vi "Generate Process.vi"(8 "error in (no error)":errorcluster, 9 "Directory":path, 10 "Name":string, 11 "Process Generator In":refnum<class "Process Generator.lvclass">) -> (0 "error out":errorcluster, 3 "Process Generator Out":refnum<class "Process Generator.lvclass">)   [LabVIEW 2020, in "Process Generator.lvclass"]
uses:
  Process Generator.lvclass
  Process Generator.lvclass/Process Generator.ctl
  Framework/Process/Process.lvclass
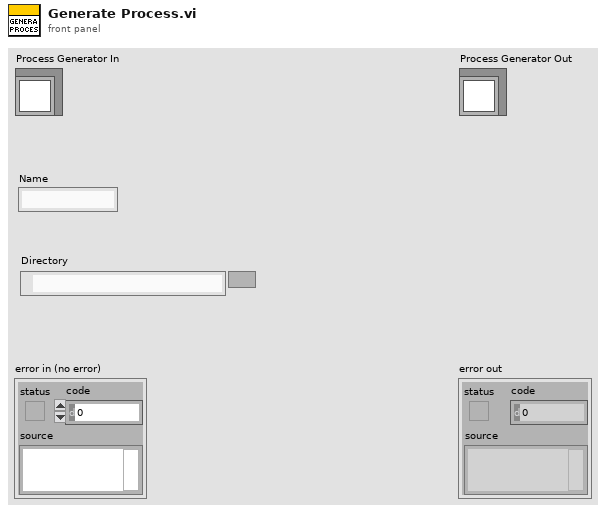
[diagram p1: front panel]
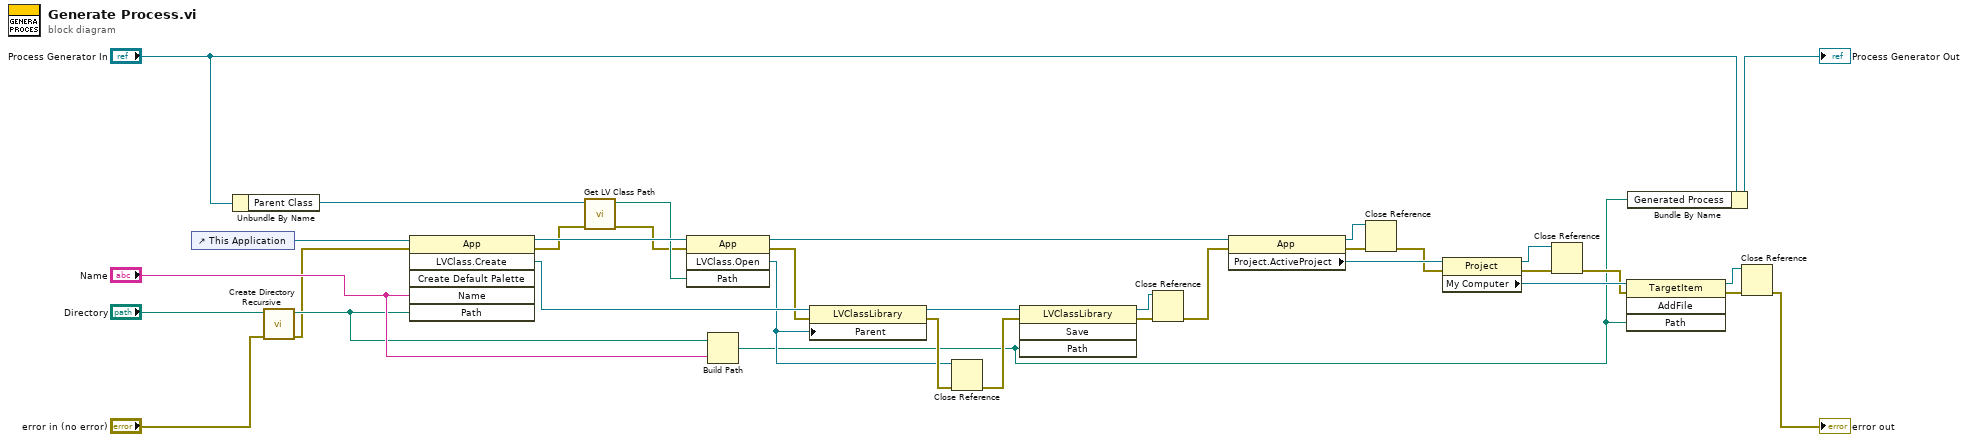
[diagram p0: block diagram]
diagram:
  n1 = control-ref of="This Application"() -> (w1:refnum<vi>)
  n2 = Unbundle By Name("Process Generator In") -> ("Parent Class"=w33:refnum<class "Process.lvclass">)
  n3 = call <vilib>:"Create Directory Recursive.vi"("error in (no error)"="error in (no error)", "directory"="Directory") -> ("error out"=w15:errorcluster, "directory copy"=w17:path)  [unwired: 3 in, 1 out]
  n4 = invoke class="App" method="LVClass.Create"(reference=w1, error in=w15, "Name"="Name", "Path"=w17) -> (reference out=w32:refnum<vi>, error out=w14:errorcluster, "LVClass.Create"=w35:refnum<vi>)  [unwired: 2 in, 3 out]
  n5 = call <vilib>:"Get LV Class Path.vi"("error in (no error)"=w14, "object"=w33) -> ("error out"=w13:errorcluster, "class path"=w31:path)  [unwired: 8 in]
  n6 = invoke class="App" method="LVClass.Open"(reference=w32, error in=w13, "Path"=w31) -> (reference out=w29:refnum<vi>, error out=w30:errorcluster, "LVClass.Open"=w4:refnum<vi>)  [unwired: 1 in, 1 out]
  n7 = Build Path(base path=w17, name or relative path="Name") -> (appended path=w2:path)
  n8 = property class="LVClassLibrary"(reference=w35, error in=w30, "Parent"=w4) -> (reference out=w25:refnum<vi>, error out=w24:errorcluster)
  n9 = Close Reference(reference=w4, error in (no error)=w24) -> (error out=w5:errorcluster)
  n10 = invoke class="LVClassLibrary" method="Save"(reference=w25, error in=w5, "Path"=w2) -> (reference out=w20:refnum<vi>, error out=w23:errorcluster)  [unwired: 1 in, 2 out]
  n11 = Close Reference(reference=w20, error in (no error)=w23) -> (error out=w21:errorcluster)
  n12 = property class="App"(reference=w29, error in=w21) -> (reference out=w11:refnum<vi>, error out=w27:errorcluster, "Project.ActiveProject"=w28:refnum<vi>)
  n13 = Close Reference(reference=w11, error in (no error)=w27) -> (error out=w12:errorcluster)
  n14 = property class="Project"(reference=w28, error in=w12) -> (reference out=w9:refnum<vi>, error out=w19:errorcluster, "My Computer"=w26:refnum<vi>)
  n15 = Close Reference(reference=w9, error in (no error)=w19) -> (error out=w10:errorcluster)
  n16 = invoke class="TargetItem" method="AddFile"(reference=w26, error in=w10, "Path"=w2) -> (reference out=w7:refnum<vi>, error out=w18:errorcluster)  [unwired: 1 in, 2 out]
  n17 = Bundle By Name(cluster="Process Generator In", "Generated Process"=w2) -> (→"Process Generator Out":refnum<class "Process Generator.lvclass">)
  n18 = Close Reference(reference=w7, error in (no error)=w18) -> (error out=→"error out":errorcluster)
